vi "get timings.vi"(8 "error in (no error)":errorcluster caption="Fehler (Eingang, kein Fehler)", 11 "TestInterface (Eingang)":refnum<class "TestInterface.lvclass">) -> (0 "error out":errorcluster caption="Fehler (Ausgang)", 2 "timings":i32[](array[numeric]), 3 "TestInterface (Ausgang)":refnum<class "TestInterface.lvclass">)   [LabVIEW 2013, in "TestInterface.lvclass"]
uses:
  TestInterface.lvclass
  TestInterface.lvclass/TestInterface.ctl
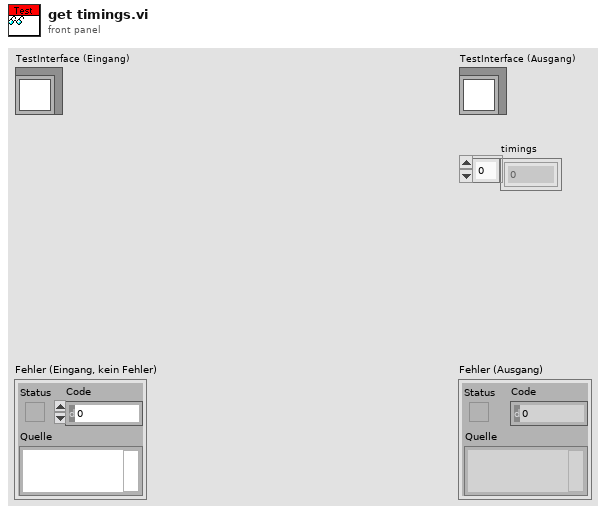
[diagram p1: front panel]
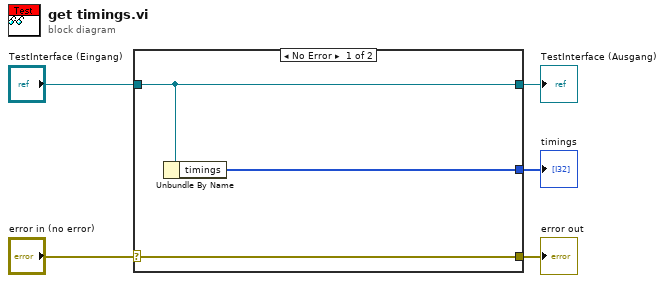
[diagram p0: block diagram]
diagram:
  n1 = case shown="No Error" "error in (no error)" {
    selector: "error in (no error)" -> [w8 w9]
    tunnel: [w8 w9] -> w4
    tunnel: [w7 w10] -> w2
    tunnel: "TestInterface (Eingang)" -> [w7 w10]
    tunnel: [w6 _] -> w1
    frame No Error {
      n2 = Unbundle By Name(w7) -> ("timings"=w6:i32[])
    }
    frame Error {
    }
  }
  "error out" <- w4
  "TestInterface (Ausgang)" <- w2
  "timings" <- w1
